vi "0.Yolov8_Condidence.vi"() -> ()   [LabVIEW 2021]
uses:
  detect_lay.dll
panel:
  out "运行时间":u32
  out "output":i32[](array[numeric])
  out "error out 2":errorcluster
  out "error out":errorcluster
  out "time(ms)":dbl
  in  "img_Path":path
  out "roi":T1(plugin-control)
  out "Original":T1(plugin-control)
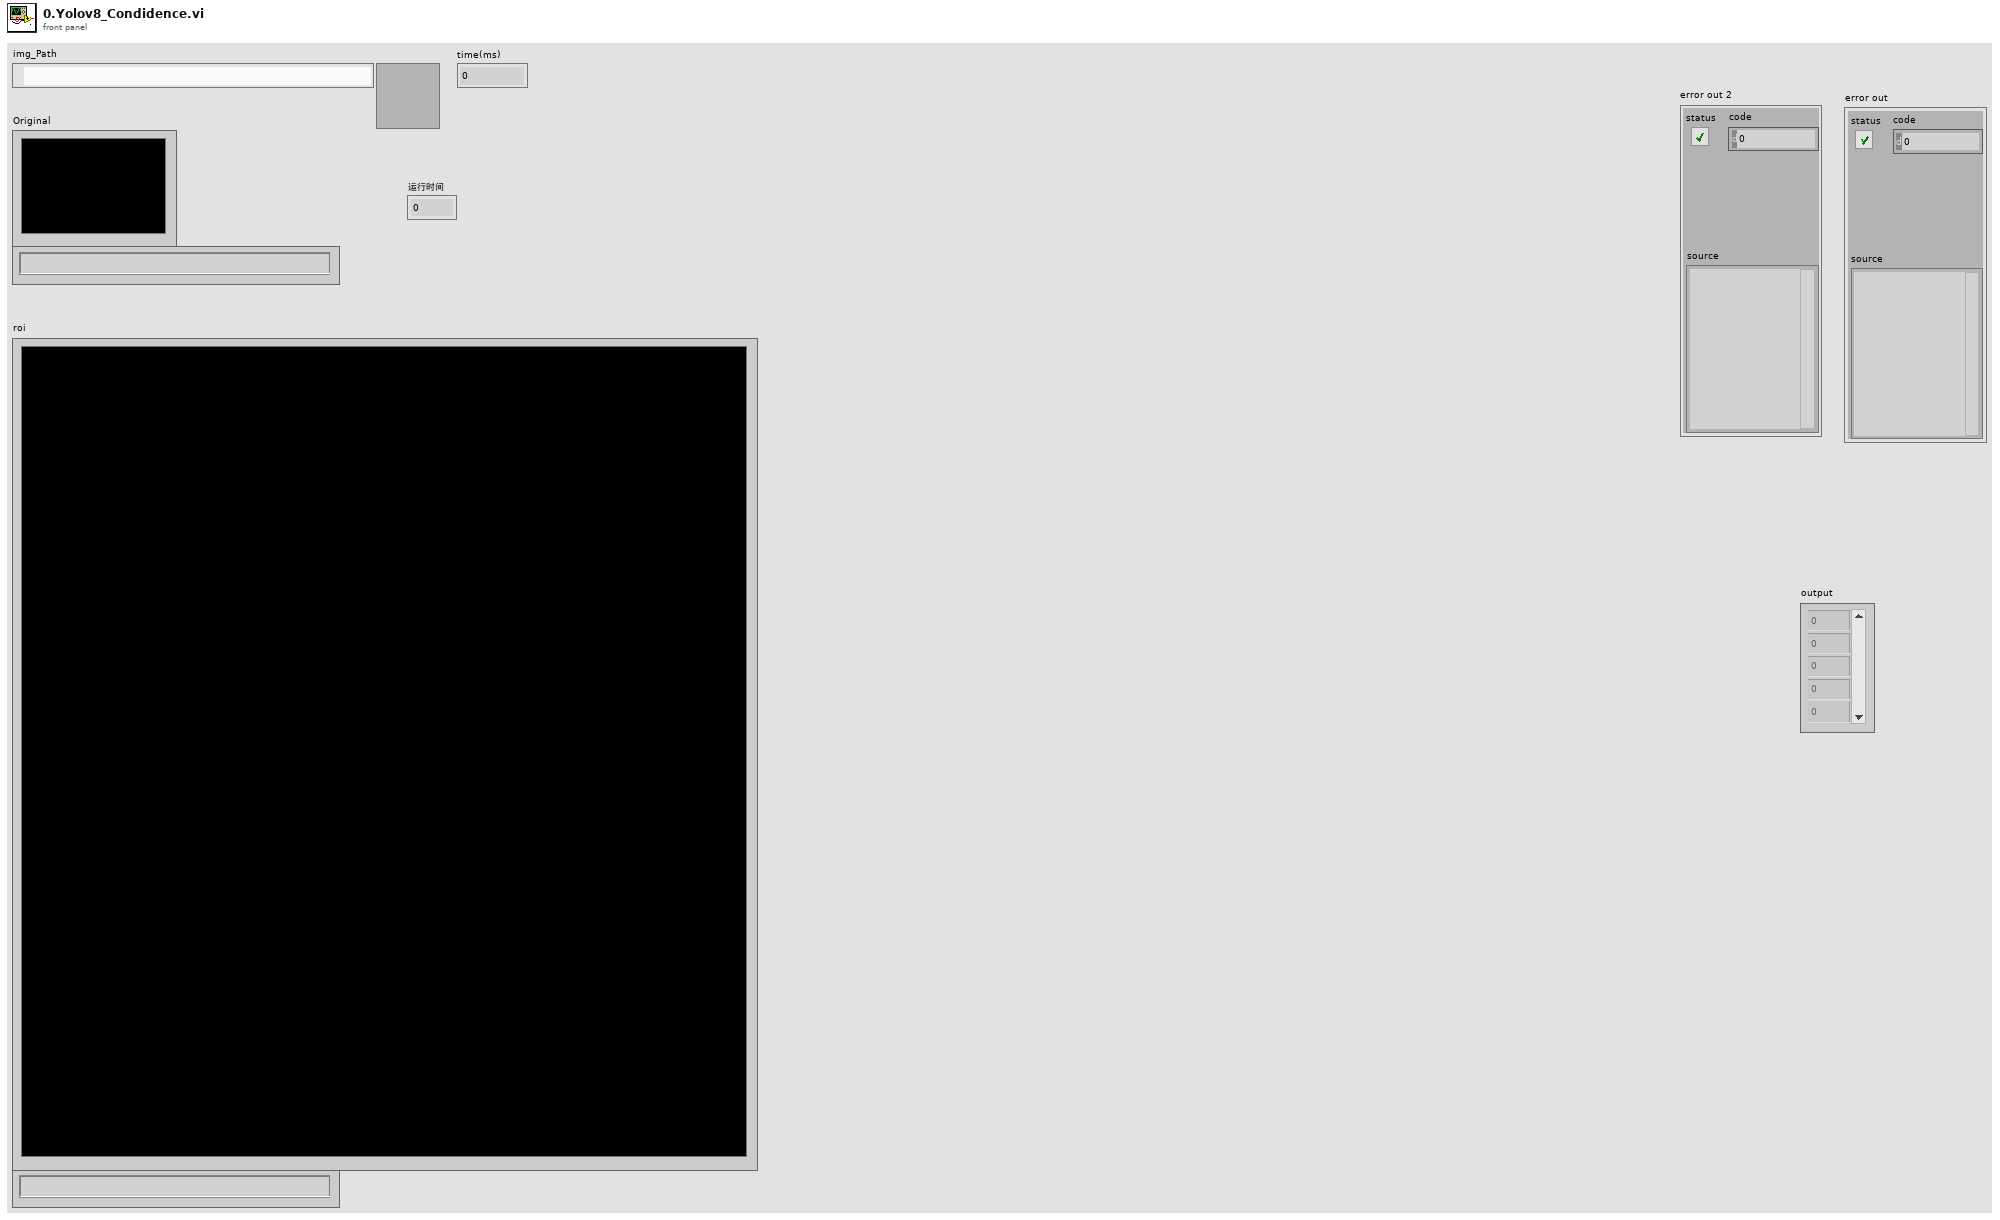
[diagram p1: front panel]
types:
  T1 = typedef "IMAQ Image.ctl" = refnum<image>
  T2 = typedef "Image Type" = u32
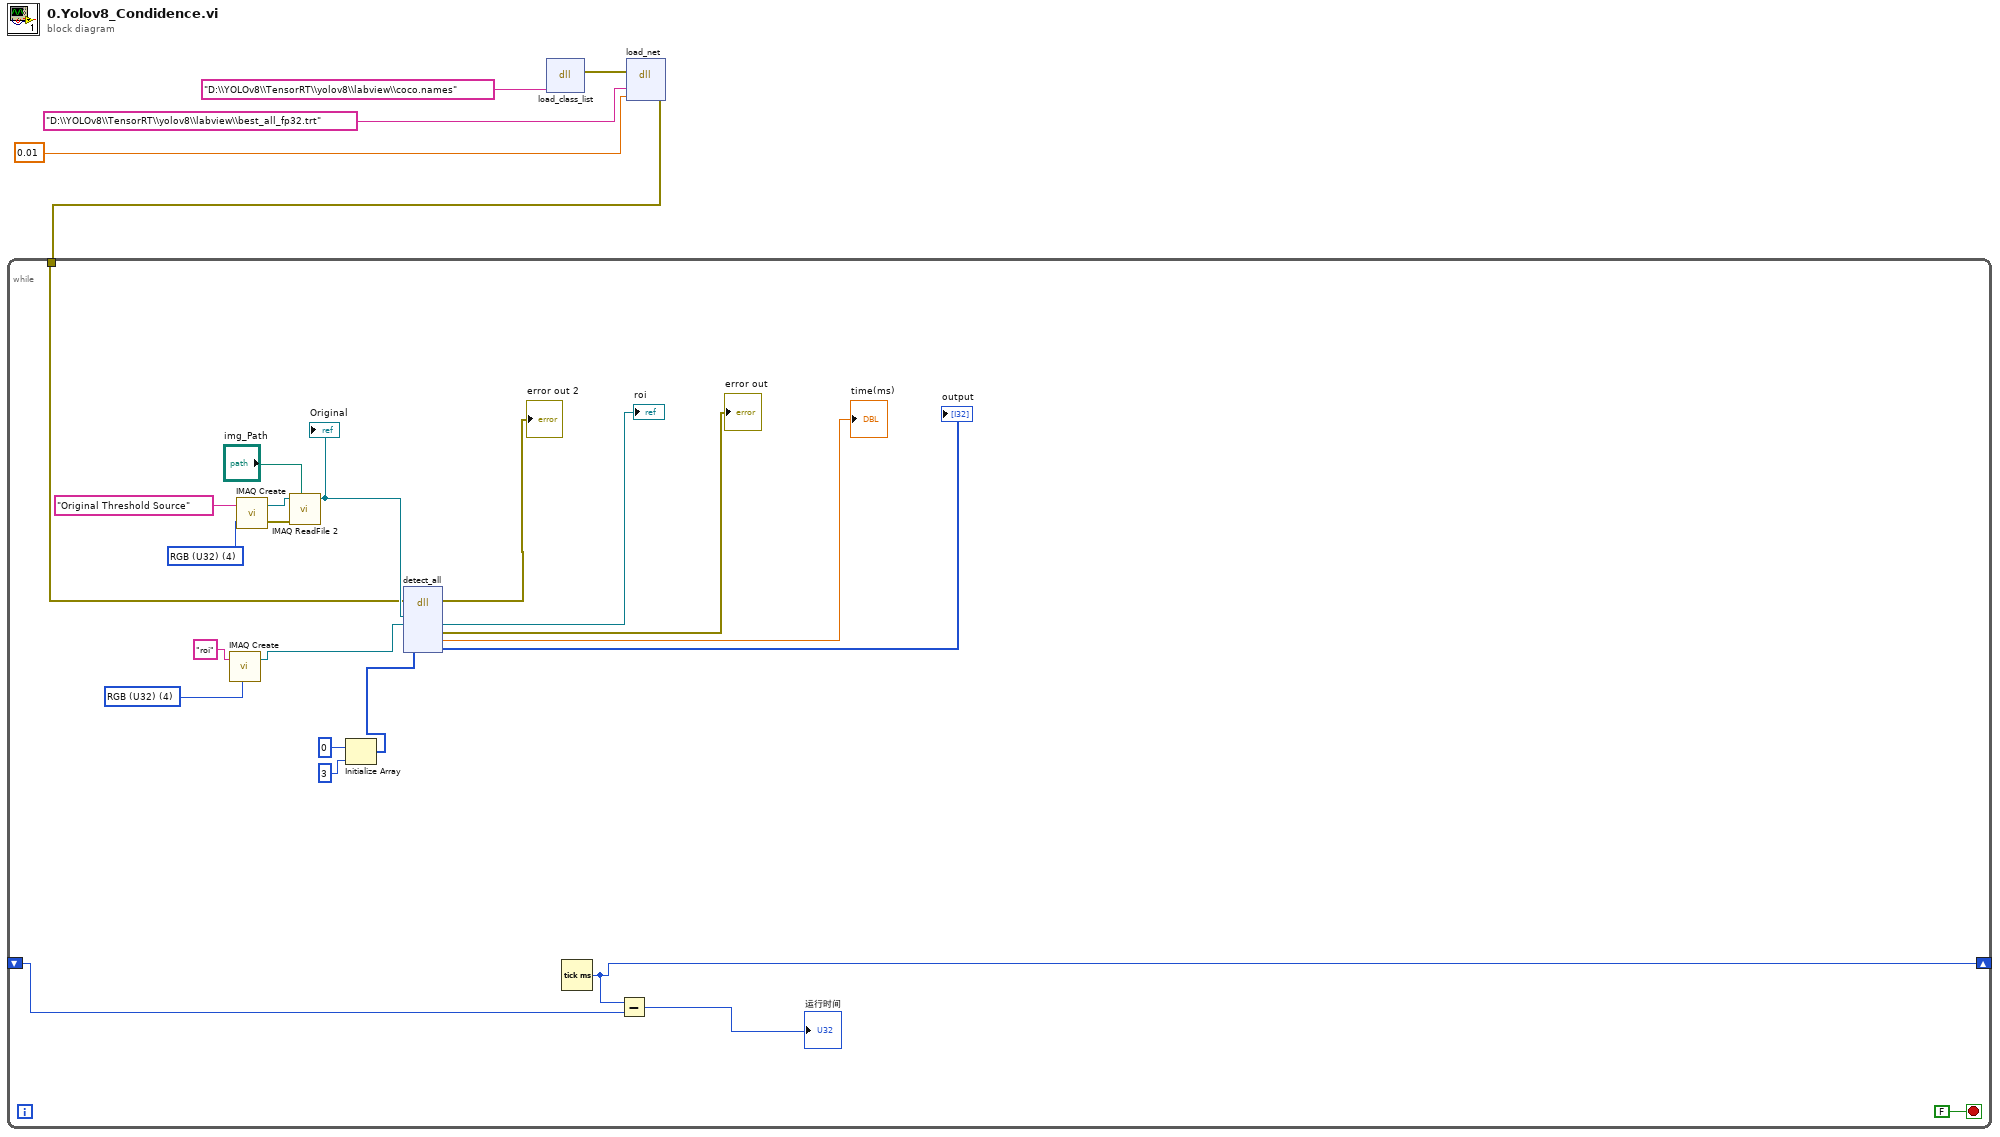
[diagram p0: block diagram]
diagram:
  n1 = dll-call lib="D:/YOLOv8/TensorRT/yolov8/labview/detect_lay.dll" fn="load_class_list"("path"="D:\\YOLOv8\\TensorRT\\yolov8\\labview\\coco.names") -> (error out=w5:errorcluster)  [unwired: 5 in, 1 out]
  n2 = dll-call lib="D:/YOLOv8/TensorRT/yolov8/labview/detect_lay.dll" fn="load_net"(error in=w5, "path"="D:\\YOLOv8\\TensorRT\\yolov8\\labview\\best_all_fp32.trt", "score_threshold"=0.01) -> (error out=w1:errorcluster)  [unwired: 5 in, 1 out]
  n3 = while {
    shift-right: [w8] -> _
    shift-left: _ -> [w9]
    tunnel: w1 -> [w6]
    stop <- FALSE stop-if-true
    w21 = T2 4 items=["Grayscale (U8)", "Grayscale (I16)", "Grayscale (SGL)", "Complex (CSG)", "RGB (U32)", "HSL (U32)", "RGB (U64)", "Grayscale (U16)"] ("Image Type")
    w24 = T2 4 items=["Grayscale (U8)", "Grayscale (I16)", "Grayscale (SGL)", "Complex (CSG)", "RGB (U32)", "HSL (U32)", "RGB (U64)", "Grayscale (U16)"] ("Image Type")
    n4 = call "IMAQ Create"("Image Name"="roi", "Image Type"=w21) -> ("New Image"=w20:T1)  [unwired: 3 in, 1 out]
    n5 = call "IMAQ Create"("Image Name"="Original Threshold Source", "Image Type"=w24) -> ("New Image"=w26:T1, "error out"=w25:errorcluster)  [unwired: 3 in]
    n6 = call "IMAQ ReadFile 2"("File Path"="img_Path", "error in (no error)"=w25, "Image"=w26) -> ("Image Out"=w11:T1)  [unwired: 4 in, 4 out]
    "Original" <- w11
    n7 = Initialize Array(0, 3) -> (w14:i32[])
    n8 = dll-call lib="D:/YOLOv8/TensorRT/yolov8/labview/detect_lay.dll" fn="detect_all"(error in=w6, "sourceHandle_src"=w11, "destHandle"=w20, "exist"=w14) -> (error out=→"error out 2":errorcluster, "destHandle"=→"roi":T1, "error out"=→"error out":errorcluster, "time"=→"time(ms)":dbl, "exist"=→"output":i32[])  [unwired: 6 in, 1 out]
    n9 = Tick Count (ms)() -> (millisecond timer value=w8:u32)
    n10 = Subtract(x=w8, y=w9) -> (x-y=→"运行时间":u32)
  }
